vi "Configure Event Action.vi"(0 "VISA resource name":refnum<visa-resource-name>, 1 "Event":T2={"Event Type (0: Internal Switch)"=0, "Event Number (1)"="1", "Event Detail (1: Alarm Level 1)"=1, "Operation Mode (0: Rising Edge)"=0} {"Event Detail (1: Alarm Level 1)" items=["Alarm Level 1"=1, "Alarm Level 2"=2, "Alarm Level 3"=3, "Alarm Level 4"=4, "Record"=5, "Computation"=6, "User Lock Out"=7, "Under Login"=8, "Memory/Media Error"=9, "Measurement Error"=10, "Communication Error"=11, "Wireless Input Unit Error"=12]; "Event Type (0: Internal Switch)" items=["Internal Switch", "Remote", "Relay", "Alarm - I/O Channel", "Alarm - Math Channel", "Alarm - Communication Channel", "Any Alarm", "Timer", "Match Time Timer", "User Function", "Status"]; "Operation Mode (0: Rising Edge)" items=["Rising Edge", "Falling Edge", "Rising / Falling Edge", "Edge"]}, 2 "Action":T1={"Action Type (0: Record)"=0, "Action Number (1)"=1, "Detail (0: start)"=0, "Group Number (1)"=1, "Batch Group Number  (0: OFF)"=0} {"Batch Group Number  (0: OFF)" items=["OFF", "1", "2", "3", "4", "5", "6", "7", "8", "9", "10", "11", "12", "ALL"]; "Group Number (1)" min=1 max=60; "Detail (0: start)" items=["Start", "Stop", "Reset", "All", "Select", "Off", "On"]; "Action Number (1)" min=1 max=6932; "Action Type (0: Record)" items=["Record", "Computation", "Manual Sample", "Alarm ACK", "Snapshot", "Adjust Time", "Save Display Data", "Save Event Data", "Event Trigger", "Message", "Switch The Display Group", "Reset The Relative Timer", "Load Config", "Show The Favorite Display", "Switch The Display Rate", "Flag", "Recording Start/Stop", "Computation Start/Stop", "Switch The Display Rate 1/2", "Flag On/Off", "Relay", "Internal Switch", "Relay On/Off", "Internal Switch On/Off", "Save Config", "Program Pattern Load"]}, 5 "No. (1)":i32=1 min=1 max=50, 7 "Enabled Event Action (Disable)":bool, 11 "error in (no error)":errorcluster) -> (4 "VISA resource name out":refnum<visa-resource-name>, 6 "No.":i32, 15 "error out":errorcluster)   [LabVIEW 2020, in "Yokogawa GX Series.lvlib"]
doc: "Sets an event action.\n\nCommand: SEventAction"
uses:
  <instrlib>/Yokogawa GX Series/Yokogawa GX Series.lvlib
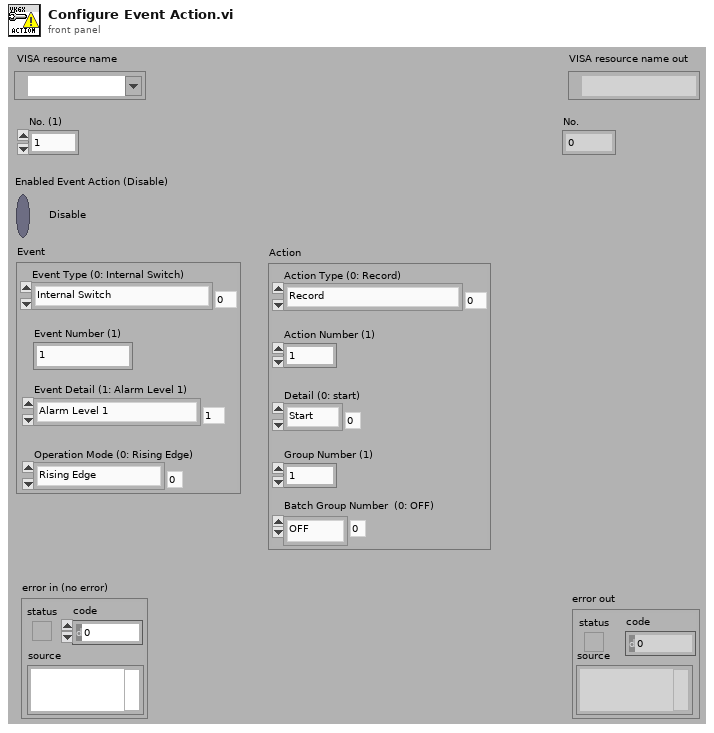
[diagram p1: front panel]
types:
  T1 = cluster{"Action Type (0: Record)":u16, "Action Number (1)":i32, "Detail (0: start)":u16, "Group Number (1)":i32, "Batch Group Number  (0: OFF)":i32}
  T2 = cluster{"Event Type (0: Internal Switch)":u16, "Event Number (1)":string, "Event Detail (1: Alarm Level 1)":i32, "Operation Mode (0: Rising Edge)":u16}
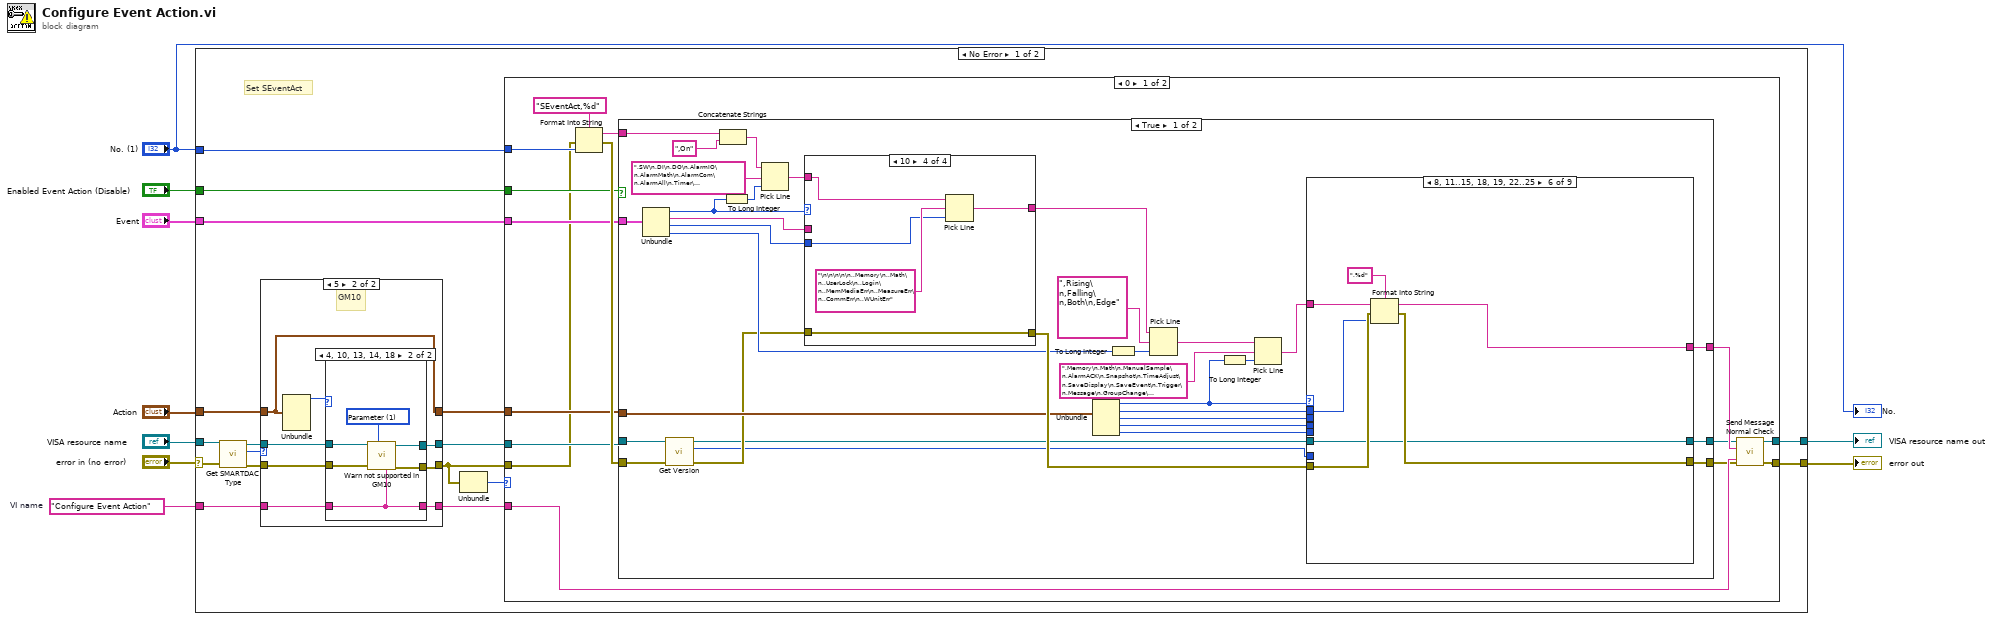
[diagram p0: block diagram]
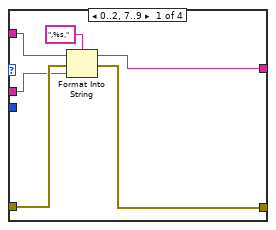
[diagram p2: hidden frame]
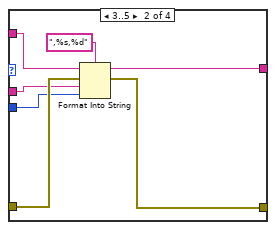
[diagram p3: hidden frame]
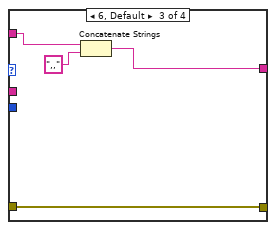
[diagram p4: hidden frame]
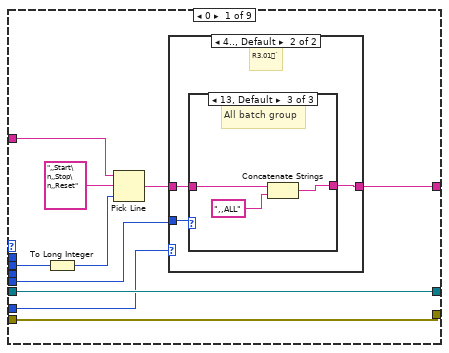
[diagram p5: hidden frame]
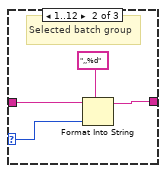
[diagram p8: hidden frame]
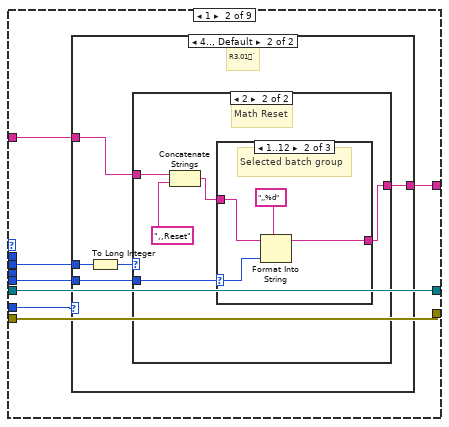
[diagram p9: hidden frame]
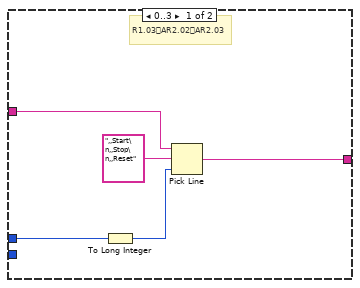
[diagram p10: hidden frame]
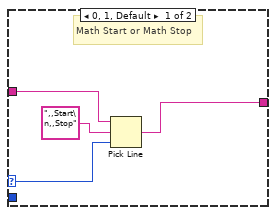
[diagram p11: hidden frame]
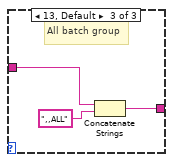
[diagram p13: hidden frame]
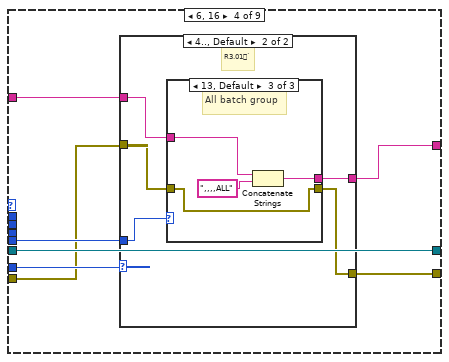
[diagram p15: hidden frame]
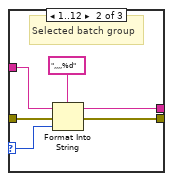
[diagram p18: hidden frame]
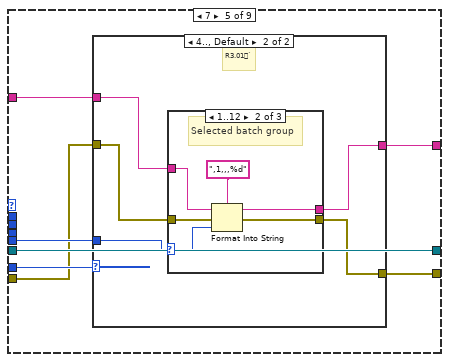
[diagram p19: hidden frame]
diagram:
  w9 = "Configure Event Action"  # VI name
  n1 = case shown="No Error" "error in (no error)" {
    selector: "error in (no error)" -> [w21 w302]
    tunnel: w9 -> [w11 _]
    tunnel: [w26 w303] -> w8
    tunnel: [w25 w302] -> w7
    tunnel: "Enabled Event Action (Disable)" -> [w24 _]
    tunnel: "No. (1)" -> [w23 _]
    tunnel: "VISA resource name" -> [w22 w303]
    tunnel: "Action" -> [w16 _]
    tunnel: "Event" -> [w12 _]
    frame No Error {
      # "Set SEventAct"
      n2 = call <instrlib>:"Get SMARTDAC Type.vi"("error in (no error)"=w21, "VISA resource name"=w22) -> ("error out"=w19:errorcluster, "SMARTDAC+ Type"=w18:u16, "VISA resource name out"=w20:refnum<visa-resource-name>)  [unwired: 7 in]
      n3 = case shown="5" w18 {
        tunnel: w20 -> [w284 w292]
        tunnel: w19 -> [w283 w291]
        tunnel: [w284 w289] -> w17
        tunnel: [w283 w288] -> w14
        tunnel: w16 -> [w282 w287]
        tunnel: [w282 w287] -> w15
        tunnel: w11 -> [w281 w286]
        tunnel: [w281 w285] -> w10
        frame 0, Default {
          # "Except GM10"
        }
        frame 5 {
          # "GM10"
          n4 = Unbundle(w287) -> ("Action Type (0: Record)"=w290:u16)  [unwired: 4 out]
          n5 = case shown="4, 10, 13, 14, 18" w290 {
            tunnel: w292 -> [w295 w301]
            tunnel: w291 -> [w294 w300]
            tunnel: [w295 w299] -> w289
            tunnel: [w294 w298] -> w288
            tunnel: w286 -> [w293 w296]
            tunnel: [w293 w296] -> w285
            frame 0, Default {
            }
            frame 4, 10, 13, 14, 18 {
              w297 = u16 1 items=["Command", "Parameter"] ("Kind (0: Command)")
              n6 = call <instrlib>:"Warn not supported in GM10.vi"("Source (\"\")"=w296, "Kind (0: Command)"=w297, "error in (no error)"=w300, "VISA resource name"=w301) -> ("error out"=w298:errorcluster, "VISA resource name out"=w299:refnum<visa-resource-name>)  [unwired: 6 in]
            }
          }
        }
      }
      n7 = Unbundle(w14) -> ("code"=w13:i32)  [unwired: 2 out]
      n8 = case shown="0" w13 {
        tunnel: w10 -> [w41 _]
        tunnel: [w40 w280] -> w26
        tunnel: [w39 w279] -> w25
        tunnel: w24 -> [w34 _]
        tunnel: w23 -> [w33 _]
        tunnel: w17 -> [w30 w280]
        tunnel: w12 -> [w29 _]
        tunnel: w15 -> [w28 _]
        tunnel: w14 -> [w27 w279]
        frame 0 {
          n9 = Format Into String(format string="SEventAct,%d", error in=w27, w33) -> (resulting string=w38:string, error out=w37:errorcluster)  [unwired: 1 in]
          n10 = case shown="True" w34 {
            tunnel: w38 -> [w74 w278]
            tunnel: w37 -> [w44 w276]
            tunnel: [w62 w276] -> w36
            tunnel: [w71 w275] -> w35
            tunnel: w30 -> [w45 w274]
            tunnel: [w61 w274] -> w32
            tunnel: w28 -> [w60 _]
            tunnel: w29 -> [w56 _]
            frame True {
              n11 = Unbundle(w56) -> ("Event Type (0: Internal Switch)"=w50:u16, "Event Number (1)"=w55:string, "Event Detail (1: Alarm Level 1)"=w54:i32, "Operation Mode (0: Rising Edge)"=w48:u16)
              n12 = call <instrlib>:"Get Version.vi"("error in (no error)"=w44, "VISA resource name"=w45) -> ("error out"=w47:errorcluster, "Version"=w43:i32, "VISA resource name out"=w46:refnum<visa-resource-name>)  [unwired: 7 in]
              n13 = Concatenate Strings(w74, ",On") -> (w69:string)
              n14 = To Long Integer(number=w50) -> (32bit integer=w51:i32)
              n15 = Pick Line(string ("")=w69, multi-line string=",SW\n,DI\n,DO\n,AlarmIO\n,AlarmMath\n,AlarmCom\n,AlarmAll\n,Timer\n,MatchTimeTimer\n,UserFunction\n,Status", line index=w51) -> (output string=w67:string)
              n16 = case shown="10" w50 {
                tunnel: w55 -> [w76 w83 _ _]
                tunnel: w54 -> [_ w82 _ w94]
                tunnel: w47 -> [w79 w87 w88 w92]
                tunnel: [w77 w81 w88 w92] -> w70
                tunnel: w67 -> [w80 w86 w90 w96]
                tunnel: [w75 w84 w89 w93] -> w63
                frame 0..2, 7..9 {
                  n17 = Format Into String(format string=",%s,", initial string=w80, error in=w79, w76) -> (resulting string=w75:string, error out=w77:errorcluster)
                }
                frame 3..5 {
                  n18 = Format Into String(format string=",%s,%d", initial string=w86, error in=w87, w83, w82) -> (resulting string=w84:string, error out=w81:errorcluster)
                }
                frame 6, Default {
                  n19 = Concatenate Strings(w90, ",,") -> (w89:string)
                }
                frame 10 {
                  n20 = Pick Line(string ("")=w96, multi-line string="\n\n\n\n\n,,Memory\n,,Math\n,,UserLock\n,,Login\n,,MemMediaErr\n,,MeasureErr\n,,CommErr\n,,WUnitErr", line index=w94) -> (output string=w93:string)
                }
              }
              n21 = Unbundle(w60) -> ("Action Type (0: Record)"=w52:u16, "Action Number (1)"=w59:i32, "Detail (0: start)"=w58:u16, "Group Number (1)"=w57:i32, "Batch Group Number  (0: OFF)"=w42:i32)
              n22 = To Long Integer(number=w48) -> (32bit integer=w49:i32)
              n23 = Pick Line(string ("")=w63, multi-line string=",Rising\n,Falling\n,Both\n,Edge", line index=w49) -> (output string=w66:string)
              n24 = To Long Integer(number=w52) -> (32bit integer=w53:i32)
              n25 = Pick Line(string ("")=w66, multi-line string=",Memory\n,Math\n,ManualSample\n,AlarmACK\n,Snapshot\n,TimeAdjust\n,SaveDisplay\n,SaveEvent\n,Trigger\n,Message\n,GroupChange\n,TimerReset\n,ConfigLoad\n,PlayList\n,RateChange\n,Flag\n,MemoryStartStop\n,MathStartStop\n,RateChange1_2\n,FlagOn_Off\n,DO\n,SW\n,DOOn_Off\n,SWOn_Off\n,ConfigSave\n,ProgPatLoad", line index=w53) -> (output string=w64:string)
              n26 = case shown="8, 11..15, 18, 19, 22..25" w52 {
                tunnel: w59 -> [_ _ _ _ _ w212 w231 w250 w271]
                tunnel: w58 -> [w102 w121 _ _ _ _ w221 _ w261]
                tunnel: w57 -> [_ _ _ _ _ _ w225 _ _]
                tunnel: w70 -> [w104 w123 w155 w156 w185 w214 w233 w252 w273]
                tunnel: [w98 w125 w154 w160 w183 w210 w219 w247 w263] -> w71
                tunnel: [w104 w123 w155 w158 w182 w211 w216 w242 w264] -> w62
                tunnel: w64 -> [w105 w124 w154 w157 w184 w209 w224 w249 w268]
                tunnel: w46 -> [w103 w122 w153 w162 w188 w208 w223 w248 w267]
                tunnel: [w103 w122 w153 w162 w188 w208 w223 w248 w267] -> w61
                tunnel: w43 -> [w100 w120 _ w161 w187 _ w218 w245 _]
                tunnel: w42 -> [w97 w119 _ w159 w186 _ w215 w244 _]
                frame 0 {
                  n27 = To Long Integer(number=w102) -> (32bit integer=w101:i32)
                  n28 = Pick Line(string ("")=w105, multi-line string=",,Start\n,,Stop\n,,Reset", line index=w101) -> (output string=w99:string)
                  n29 = case shown="4.., Default" w100 {
                    tunnel: w99 -> [w107 w110]
                    tunnel: [w107 w109] -> w98
                    tunnel: w97 -> [_ w108]
                    frame 0..3 {
                      # "R1.03AR2.02AR2.03"
                    }
                    frame 4.., Default {
                      # "R3.01`"
                      n30 = case shown="13, Default" w108 {
                        selector: w108 -> [_ w112 _]
                        tunnel: w110 -> [w111 w115 w118]
                        tunnel: [w111 w113 w117] -> w109
                        frame 0 {
                          # "/BT Invalid"
                        }
                        frame 1..12 {
                          # "Selected batch group"
                          n31 = Format Into String(format string=",,%d", initial string=w115, w112) -> (resulting string=w113:string)  [unwired: 1 in, 1 out]
                        }
                        frame 13, Default {
                          # "All batch group"
                          n32 = Concatenate Strings(w118, ",,ALL") -> (w117:string)
                        }
                      }
                    }
                  }
                }
                frame 1 {
                  n33 = case shown="4.., Default" w120 {
                    tunnel: [w128 w135] -> w125
                    tunnel: w124 -> [w126 w134]
                    tunnel: w121 -> [w127 w133]
                    tunnel: w119 -> [_ w131]
                    frame 0..3 {
                      # "R1.03AR2.02AR2.03"
                      n34 = To Long Integer(number=w127) -> (32bit integer=w129:i32)
                      n35 = Pick Line(string ("")=w126, multi-line string=",,Start\n,,Stop\n,,Reset", line index=w129) -> (output string=w128:string)
                    }
                    frame 4.., Default {
                      # "R3.01`"
                      n36 = To Long Integer(number=w133) -> (32bit integer=w132:i32)
                      n37 = case shown="2" w132 {
                        selector: w132 -> [w138 _]
                        tunnel: [w136 w140] -> w135
                        tunnel: w134 -> [w137 w144]
                        tunnel: w131 -> [_ w142]
                        frame 0, 1, Default {
                          # "Math Start or Math Stop"
                          n38 = Pick Line(string ("")=w137, multi-line string=",,Start\n,,Stop", line index=w138) -> (output string=w136:string)
                        }
                        frame 2 {
                          # "Math Reset"
                          n39 = Concatenate Strings(w144, ",,Reset") -> (w141:string)
                          n40 = case shown="1..12" w142 {
                            selector: w142 -> [_ w147 _]
                            tunnel: [w145 w148 w152] -> w140
                            tunnel: w141 -> [w145 w146 w151]
                            frame 0 {
                              # "/BT Invalid"
                            }
                            frame 1..12 {
                              # "Selected batch group"
                              n41 = Format Into String(format string=",,%d", initial string=w146, w147) -> (resulting string=w148:string)  [unwired: 1 in, 1 out]
                            }
                            frame 13, Default {
                              # "All batch group"
                              n42 = Concatenate Strings(w151, ",,ALL") -> (w152:string)
                            }
                          }
                        }
                      }
                    }
                  }
                }
                frame 2..5, 17, Default {
                }
                frame 6, 16 {
                  n43 = case shown="4.., Default" w161 {
                    tunnel: w157 -> [w164 w168]
                    tunnel: [w164 w169] -> w160
                    tunnel: w159 -> [_ w167]
                    tunnel: w156 -> [w163 w166]
                    tunnel: [w163 w165] -> w158
                    frame 0..3 {
                      # "R1.03AR2.02AR2.03"
                    }
                    frame 4.., Default {
                      # "R3.01`"
                      n44 = case shown="13, Default" w167 {
                        selector: w167 -> [_ w175 _]
                        tunnel: [w171 w176 w181] -> w169
                        tunnel: w168 -> [w171 w174 w180]
                        tunnel: w166 -> [w170 w173 w178]
                        tunnel: [w170 w172 w178] -> w165
                        frame 0 {
                          # "/BT Invalid"
                        }
                        frame 1..12 {
                          # "Selected batch group"
                          n45 = Format Into String(format string=",,,,%d", initial string=w174, error in=w173, w175) -> (resulting string=w176:string, error out=w172:errorcluster)
                        }
                        frame 13, Default {
                          # "All batch group"
                          n46 = Concatenate Strings(w180, ",,,,ALL") -> (w181:string)
                        }
                      }
                    }
                  }
                }
                frame 7 {
                  n47 = case shown="4.., Default" w187 {
                    tunnel: w184 -> [w190 w193]
                    tunnel: w186 -> [_ w192]
                    tunnel: w185 -> [w189 w194]
                    tunnel: [w190 w191] -> w183
                    tunnel: [w189 w195] -> w182
                    frame 0..3 {
                      # "R1.03AR2.02AR2.03"
                    }
                    frame 4.., Default {
                      # "R3.01`"
                      n48 = case shown="1..12" w192 {
                        selector: w192 -> [_ w202 _]
                        tunnel: [w197 w203 w207] -> w191
                        tunnel: w193 -> [w197 w201 w206]
                        tunnel: w194 -> [w196 w200 w204]
                        tunnel: [w196 w199 w204] -> w195
                        frame 0 {
                          # "/BT Invalid"
                        }
                        frame 1..12 {
                          # "Selected batch group"
                          n49 = Format Into String(format string=",1,,,%d", initial string=w201, error in=w200, w202) -> (resulting string=w203:string, error out=w199:errorcluster)
                        }
                        frame 13, Default {
                          # "All batch group"
                          n50 = Concatenate Strings(w206, ",1,,,ALL") -> (w207:string)
                        }
                      }
                    }
                  }
                }
                frame 8, 11..15, 18, 19, 22..25 {
                  n51 = Format Into String(format string=",%d", initial string=w209, error in=w214, w212) -> (resulting string=w210:string, error out=w211:errorcluster)
                }
                frame 9 {
                  n52 = Format Into String(format string=",%d", initial string=w224, error in=w233, w231) -> (resulting string=w230:string, error out=w227:errorcluster)
                  n53 = To Long Integer(number=w221) -> (32bit integer=w222:i32)
                  n54 = Pick Line(string ("")=w230, multi-line string=",\n,\n,\n,All\n,Select", line index=w222) -> (output string=w228:string)
                  n55 = Format Into String(format string=",%d", initial string=w228, error in=w227, w225) -> (resulting string=w220:string, error out=w217:errorcluster)
                  n56 = case shown="4.., Default" w218 {
                    tunnel: [w235 w240] -> w219
                    tunnel: w220 -> [w235 w239]
                    tunnel: w217 -> [w234 w238]
                    tunnel: [w234 w237] -> w216
                    tunnel: w215 -> [_ w236]
                    frame 0..3 {
                      # "R1.03AR2.02AR2.03"
                    }
                    frame 4.., Default {
                      # "R3.01`"
                      n57 = Format Into String(format string=",%d", initial string=w239, error in=w238, w236) -> (resulting string=w240:string, error out=w237:errorcluster)
                    }
                  }
                }
                frame 10 {
                  n58 = Format Into String(format string=",%d", initial string=w249, error in=w252, w250) -> (resulting string=w246:string, error out=w243:errorcluster)
                  n59 = case shown="4.., Default" w245 {
                    tunnel: [w254 w259] -> w247
                    tunnel: w246 -> [w254 w258]
                    tunnel: w244 -> [_ w257]
                    tunnel: w243 -> [w253 w256]
                    tunnel: [w253 w255] -> w242
                    frame 0..3 {
                      # "R1.03AR2.02AR2.03"
                    }
                    frame 4.., Default {
                      # "R3.01`"
                      n60 = Format Into String(format string=",,,%d", initial string=w258, error in=w256, w257) -> (resulting string=w259:string, error out=w255:errorcluster)
                    }
                  }
                }
                frame 20, 21 {
                  n61 = Format Into String(format string=",%d", initial string=w268, error in=w273, w271) -> (resulting string=w270:string, error out=w264:errorcluster)
                  n62 = To Long Integer(number=w261) -> (32bit integer=w262:i32)
                  n63 = Subtract(x=w262, y=5) -> (x-y=w265:i32)
                  n64 = Pick Line(string ("")=w270, multi-line string=",Off\n,On", line index=w265) -> (output string=w263:string)
                }
              }
            }
            frame False {
              n65 = Concatenate Strings(w278, ",Off") -> (w275:string)
            }
          }
          n66 = call <instrlib>:"Send Message Normal Check.vi"("Source (\"\")"=w41, "error in (no error)"=w36, "Send Message (\"\")"=w35, "VISA resource name"=w32) -> ("error out"=w39:errorcluster, "VISA resource name out"=w40:refnum<visa-resource-name>)  [unwired: 2 in, 4 out]
        }
        frame 1, Default {
        }
      }
    }
    frame Error {
    }
  }
  "error out" <- w7
  "VISA resource name out" <- w8
  "No." <- "No. (1)"
